vi "getRegularExpression.vi"(8 "error in (no error)":errorcluster, 11 "tBSONRegEx in":refnum<class "tBSONRegEx.lvclass">) -> (0 "error out":errorcluster, 2 "RegularExpression":string, 3 "tBSONRegEx out":refnum<class "tBSONRegEx.lvclass">)   [LabVIEW 2013, in "BSON.lvlib" / "tBSONRegEx.lvclass"]
uses:
  tBSONRegEx.lvclass
  tBSONRegEx.lvclass/tBSONRegEx.ctl
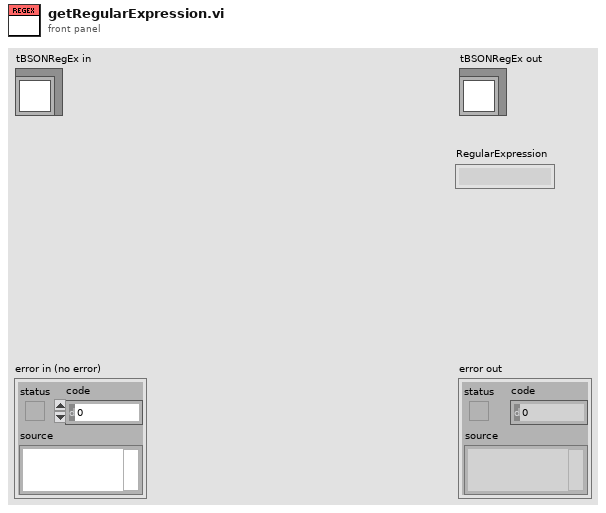
[diagram p1: front panel]
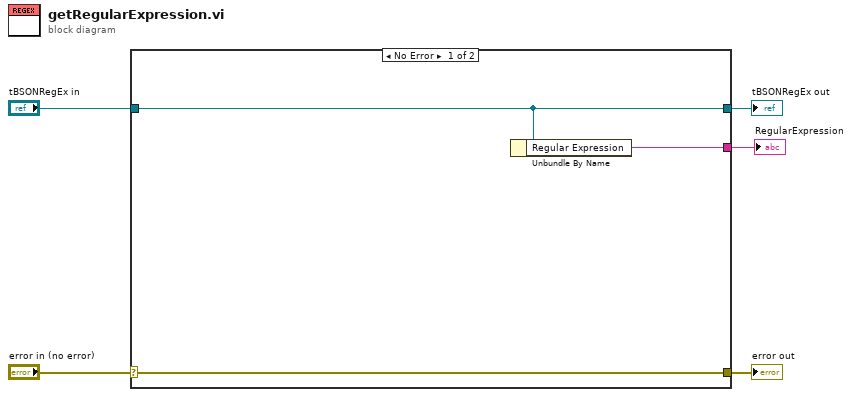
[diagram p0: block diagram]
diagram:
  n1 = case shown="No Error" "error in (no error)" {
    selector: "error in (no error)" -> [w8 w10]
    tunnel: [w8 w10] -> w4
    tunnel: [w7 w9] -> w2
    tunnel: "tBSONRegEx in" -> [w7 w9]
    tunnel: [w6 _] -> w1
    frame No Error {
      n2 = Unbundle By Name(w7) -> ("Regular Expression"=w6:string)
    }
    frame Error {
    }
  }
  "error out" <- w4
  "tBSONRegEx out" <- w2
  "RegularExpression" <- w1
